vi "GDX_ACC_ComputePitchRoll.vi"(8 "Measurements In":dbl[][](array[numeric]), 9 "dt":dbl, 10 "Gyro Percent of Filter":dbl(slide)=75.0 scale=0.0..100.0, 11 "Initialize":bool) -> (0 "Filtered Roll":dbl, 1 "Filtered Pitch":dbl, 2 "Gyro Roll":dbl, 3 "Gyro Pitch":dbl, 5 "Accel Roll":dbl, 7 "Accel Pitch":dbl)   [LabVIEW 2019]
panel:
  out "Gyro X Radians (Roll)":dbl
  out "Gyro Y Radians (Pitch)":dbl
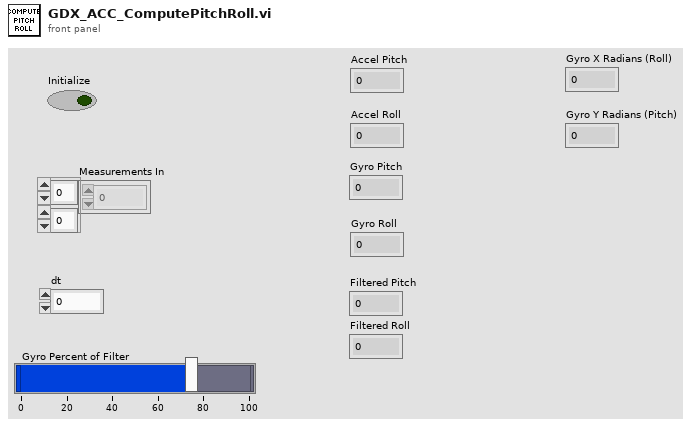
[diagram p1: front panel]
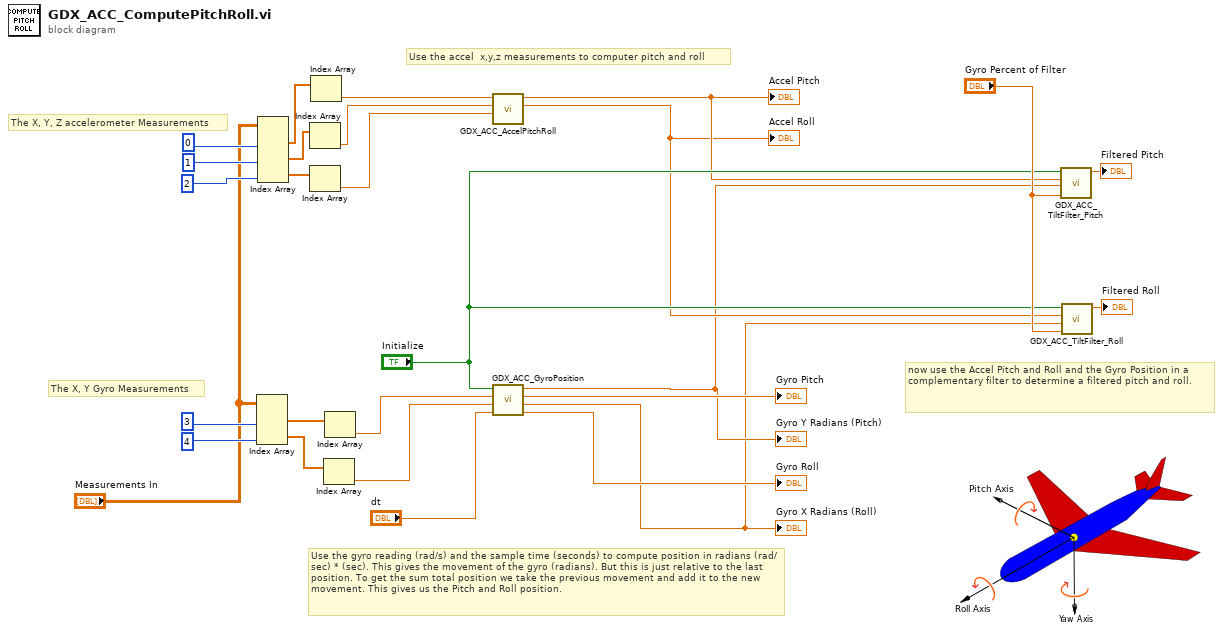
[diagram p0: block diagram]
diagram:
  # "now use the Accel Pitch and Roll and the Gyro Position in a complementary filter to determine a filtered pitch and roll."
  # "Use the gyro reading (rad/s) and the sample time (seconds) to compute position in radians (rad/sec) * (sec). This gives the movement of the gyro (radians). But this is just relative to the last position. To get the sum total position we take the previous movement and add it to the new movement. This gives us the Pitch and Roll position."
  # "Use the accel  x,y,z measurements to computer pitch and roll"
  # "The X, Y Gyro Measurements"
  # "The X, Y, Z accelerometer Measurements"
  n1 = Index Array(array="Measurements In", index (col) #1=3 ("disabled index (col)"), index (col) #2=4 ("index (col)")) -> (element #1=w23:dbl[], element #2=w24:dbl[])  [unwired: 2 in]
  n2 = Index Array(array="Measurements In", index (col) #1=0 ("disabled index (col)"), index (col) #2=1 ("index (col)"), index (col) #3=2 ("index (col)")) -> (element #1=w17:dbl[], element #2=w18:dbl[], element #3=w19:dbl[])  [unwired: 3 in]
  n3 = Index Array(array=w18) -> (element=w21:dbl)  [unwired: 1 in]
  n4 = Index Array(array=w19) -> (element=w22:dbl)  [unwired: 1 in]
  n5 = Index Array(array=w17) -> (element=w20:dbl)  [unwired: 1 in]
  n6 = Index Array(array=w24) -> (element=w27:dbl)  [unwired: 1 in]
  n7 = Index Array(array=w23) -> (element=w26:dbl)  [unwired: 1 in]
  n8 = call "GDX_ACC_AccelPitchRoll.vi"("z Accel"=w22, "y Accel"=w21, "x Accel"=w20) -> ("Roll"=w7:dbl, "Pitch"=w8:dbl)  [unwired: 7 in]
  "Accel Pitch" <- w8
  "Accel Roll" <- w7
  n9 = call "GDX_ACC_GyroPosition.vi"("dt"="dt", "Y Gyro (rad/s)"=w27, "X Gyro (rad/s)"=w26, "Initialize"="Initialize") -> ("GyroX Roll"=→"Gyro Roll":dbl, "GyroX Radians (Roll)"=w1:dbl, "GyroY Pitch"=→"Gyro Pitch":dbl, "GyroY Radians (Pitch)"=w2:dbl)  [unwired: 4 in]
  "Gyro Y Radians (Pitch)" <- w2
  "Gyro X Radians (Roll)" <- w1
  n10 = call "GDX_ACC_TiltFilter_Pitch.vi"("Gyro Percent"="Gyro Percent of Filter", "Gyro Pitch (rad)"=w2, "Accelerometer Pitch (rad)"=w8, "initialize"="Initialize") -> ("Filtered Pitch"=→"Filtered Pitch":dbl)  [unwired: 7 in]
  n11 = call "GDX_ACC_TiltFilter_Roll.vi"("Gyro Percent"="Gyro Percent of Filter", "Gyro Roll (rad)"=w1, "Accelerometer Roll (rad)"=w7, "initialize"="Initialize") -> ("Filtered Roll"=→"Filtered Roll":dbl)  [unwired: 7 in]
